vi "Default Pie Property.vi"(11 "Plot ID":i32) -> (3 "Default Property":T1)   [LabVIEW 2017, in "3D Pie.lvclass"]
uses:
  <vilib>/Math Plots/3D Math Plots/3D Pie/3D Pie/3D Pie.lvclass
  <vilib>/Math Plots/3D Math Plots/3D Pie/3D Pie/Typedef/3D Pie Property.ctl
  <vilib>/Math Plots/3D Math Plots/3D Plot/3D Plot/Typedef/Line Type.ctl
  <vilib>/Math Plots/3D Math Plots/3D Plot/3D Plot/3D Plot.lvclass
panel:
  in  "Name Prefix":string="Plot "
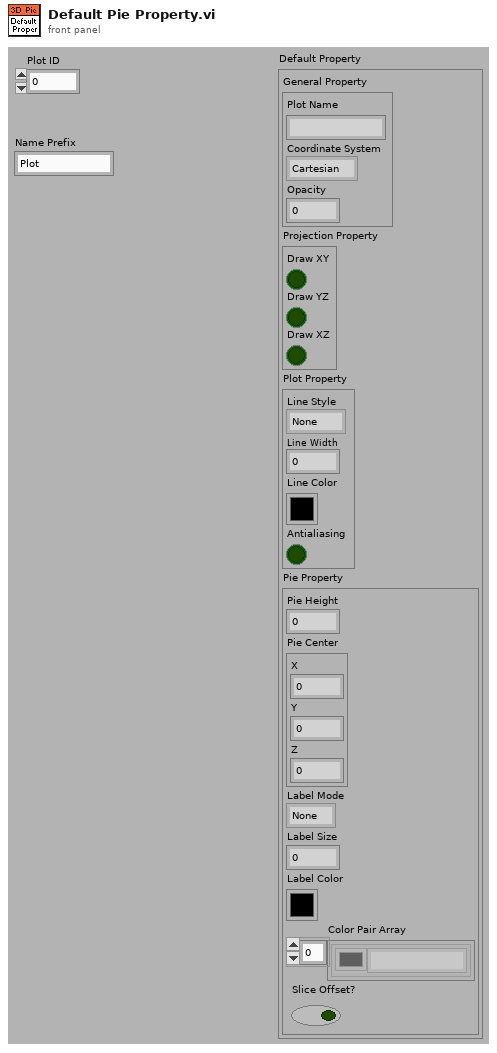
[diagram p1: front panel]
types:
  T1 = typedef "3D Pie.lvclass/3D Pie Property.ctl" = cluster{"General Property":cluster{"Plot Name":string, "Coordinate System":enum16{"Cartesian", "Cylindrical", "Spherical"}, "Opacity":sgl}, "Projection Property":cluster{"Draw XY":bool, "Draw YZ":bool, "Draw XZ":bool}, "Plot Property":cluster{"Line Style":T2, "Line Width":sgl, "Line Color":u32, "Antialiasing":bool}, "Pie Property":cluster{"Pie Height":sgl, "Pie Center":cluster{"X":sgl, "Y":sgl, "Z":sgl}, "Label Mode":enum16{"None", "Show Percentage", "Show String"}, "Label Size":u16, "Label Color":u32, "Color Pair Array":cluster{"Color":u32, "String":string}[], "Slice Offset?":bool}}
  T2 = typedef "3D Plot.lvclass/Line Type.ctl" = enum16{"None", "Solid", "Dash", "Dot", "Dash Dot"}
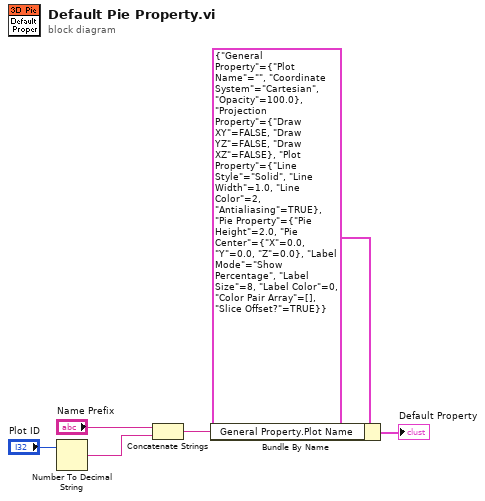
[diagram p0: block diagram]
diagram:
  n1 = Number To Decimal String(number="Plot ID") -> (decimal integer string=w6:string)  [unwired: 1 out]
  n2 = Concatenate Strings("Name Prefix", w6) -> (w3:string)
  n3 = Bundle By Name(cluster=T1 {"General Property"={"Plot Name"="", "Coordinate System"=enum."Cartesian", "Opacity"=100.0}, "Projection Property"={"Draw XY"=FALSE, "Draw YZ"=FALSE, "Draw XZ"=FALSE}, "Plot Property"={"Line Style"=enum."Solid", "Line Width"=1.0, "Line Color"=2, "Antialiasing"=TRUE}, "Pie Property"={"Pie Height"=2.0, "Pie Center"={"X"=0.0, "Y"=0.0, "Z"=0.0}, "Label Mode"=enum."Show Percentage", "Label Size"=8, "Label Color"=0, "Color Pair Array"=[], "Slice Offset?"=TRUE}} ("new element/subarray"), "General Property.Plot Name"=w3) -> (→"Default Property":T1)
